vi "Main.vi"(11 "Module Admin":refnum<class "Delacor_lib_QMH_Module Admin.lvclass">) -> ()   [LabVIEW 2020, in "Configuration.lvlib"]
doc: "This template is based off of the Queued Message Handler design pattern and the Queued Message Handler project template that ships with LabVIEW.\n\nThe main difference is that the queue is private to this module and communication between modules is performed via Broadcast and Request events.\n\nRequest events are wrapped in public API methods and are handled in the Event Handling Loop (EHL) of this VI. Any module can register for Broadcast events sent by this module. The EHL generates messages based on user interface actions.\n\nThe Message Handling Loop (MHL) processes messages generated by the EHL, or by other messages. The messages are string values, so new messages can be added easily to the Message Cases case structure in the MHL. Each message cluster can also provide an optional value for Message Data, which is a variant that can be converted to whatever message-specific data is required.\n_____\nBased on DQMH Project Template 6.1.0.94."
uses:
  Configuration.lvlib
  <vilib>/Delacor/Delacor QMH/Libraries/Module Admin_class/Delacor_lib_QMH_Module Admin.lvclass
  Module Data--cluster.ctl
  <vilib>/Delacor/Delacor QMH/Libraries/Message Queue_class/Delacor_lib_QMH_Message Queue.lvclass/Delacor_lib_QMH_Message Queue.ctl
  Stop Argument--cluster.ctl
  <vilib>/Delacor/Delacor QMH/Libraries/Module Admin_class/Delacor_lib_QMH_Module Admin.lvclass/Delacor_lib_QMH_Module Admin.ctl
  Write config Argument--cluster.ctl
  Config data.ctl
  Set config path Argument--cluster.ctl
  Load config Argument--cluster.ctl
  Load config (Reply Payload)--cluster.ctl
  <vilib>/Utility/miscctls.llb/LVPointTypeDef.ctl
  <vilib>/Delacor/Delacor QMH/Libraries/Message Queue_class/Delacor_lib_QMH_Enqueue Message (Single).vi
  <vilib>/Delacor/Delacor QMH/Libraries/Module Admin_class/Delacor_lib_QMH_Get External Launch.vi
  <vilib>/Utility/error.llb/Error Cluster From Error Code.vi
  <vilib>/Utility/config.llb/Write Key (Double).vi
  <vilib>/Utility/config.llb/Read Key (Double).vi
  <vilib>/ErrorRing/Error Ring.xnode
  <vilib>/Delacor/Delacor QMH/Libraries/Message Queue_class/Delacor_lib_QMH_Message Queue.lvclass
  <vilib>/Utility/config.llb/Read Key (String).vi
  <vilib>/Utility/config.llb/Write Key (String).vi
  <vilib>/Utility/config.llb/NI_LVConfig.lvlib
panel:
  out "error out":errorcluster
  out "Status":string
  in  "Simulate MHL Error":bool
  in  "Simulate EHL Error":bool
  # "Other QMH Modules communicate with this Module via its Public API (wrappers for its Request Events).\n\nThis Module communicates with other Modules via its Broadcast Events.\nAny module that wants to get these messages, just registers for this module's Broadcast events."
  # "This template is for the Delacor Modified Queued Message Handler design pattern.\n\nSee the block diagram for more information on how to use this template."
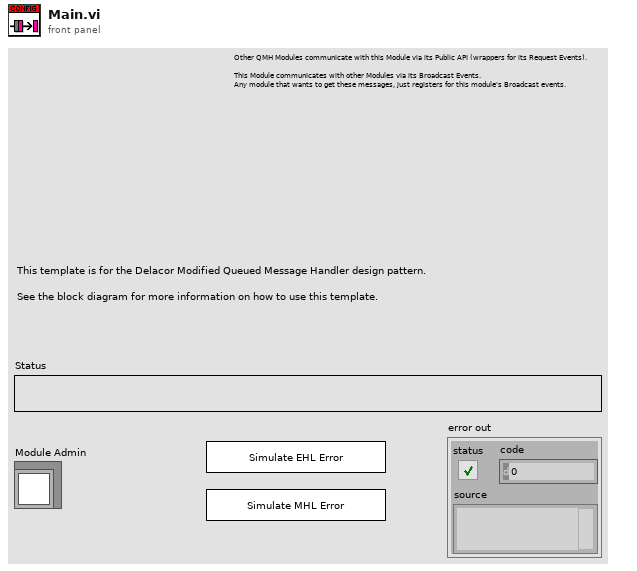
[diagram p1: front panel]
types:
  T1 = typedef "Configuration.lvlib/Request Events--cluster.ctl" = cluster{"Stop Module":refnum<user-event>, "Show Panel":refnum<user-event>, "Hide Panel":refnum<user-event>, "Get Module Execution Status":refnum<user-event>, "Show Diagram":refnum<user-event>, "Write config":refnum<user-event>, "Set config path":refnum<user-event>, "Load config":refnum<user-event>}
  T2 = typedef "Configuration.lvlib/Module Data--cluster.ctl" = cluster{"Status":string, "Config path":path}
  T3 = enum32{"invalid lock state", "Not Locked", "Locked (No Password)", "Password-protected"}
  T4 = typedef "Configuration.lvlib/Stop Argument--cluster.ctl" = cluster{"Origin":string, "Exit via Stop Module Req?":bool, "Wait for Module to stop?":bool}
  T5 = typedef "Configuration.lvlib/Write config Argument--cluster.ctl" = cluster{"Config path":path, "Data":T6}
  T6 = typedef "Configuration.lvlib/Config data.ctl" = cluster{"Arduino":string, "Steps per rev":dbl, "Config path":path, "Pitch":dbl, "Osciloscopio":refnum<visa-resource-name>}
  T7 = typedef "Configuration.lvlib/Set config path Argument--cluster.ctl" = cluster{"Config path":path}
  T8 = typedef "Configuration.lvlib/Load config Argument--cluster.ctl" = cluster{"Wait Notifier":refnum<notifier>, "wait for reply":bool}
  T9 = typedef "LVPointTypeDef.ctl" = cluster{"Horizontal":i16, "Vertical":i16}
  T10 = enum32{"Invalid", "Standard", "Closed", "Hidden", "Minimized", "Maximized"}
  T11 = typedef "Configuration.lvlib/Load config (Reply Payload)--cluster.ctl" = cluster{"Data":T6, "error":errorcluster}
  T12 = typedef "NI_LVConfig.lvlib/Config Data RefNum.ctl" = refnum<k1>
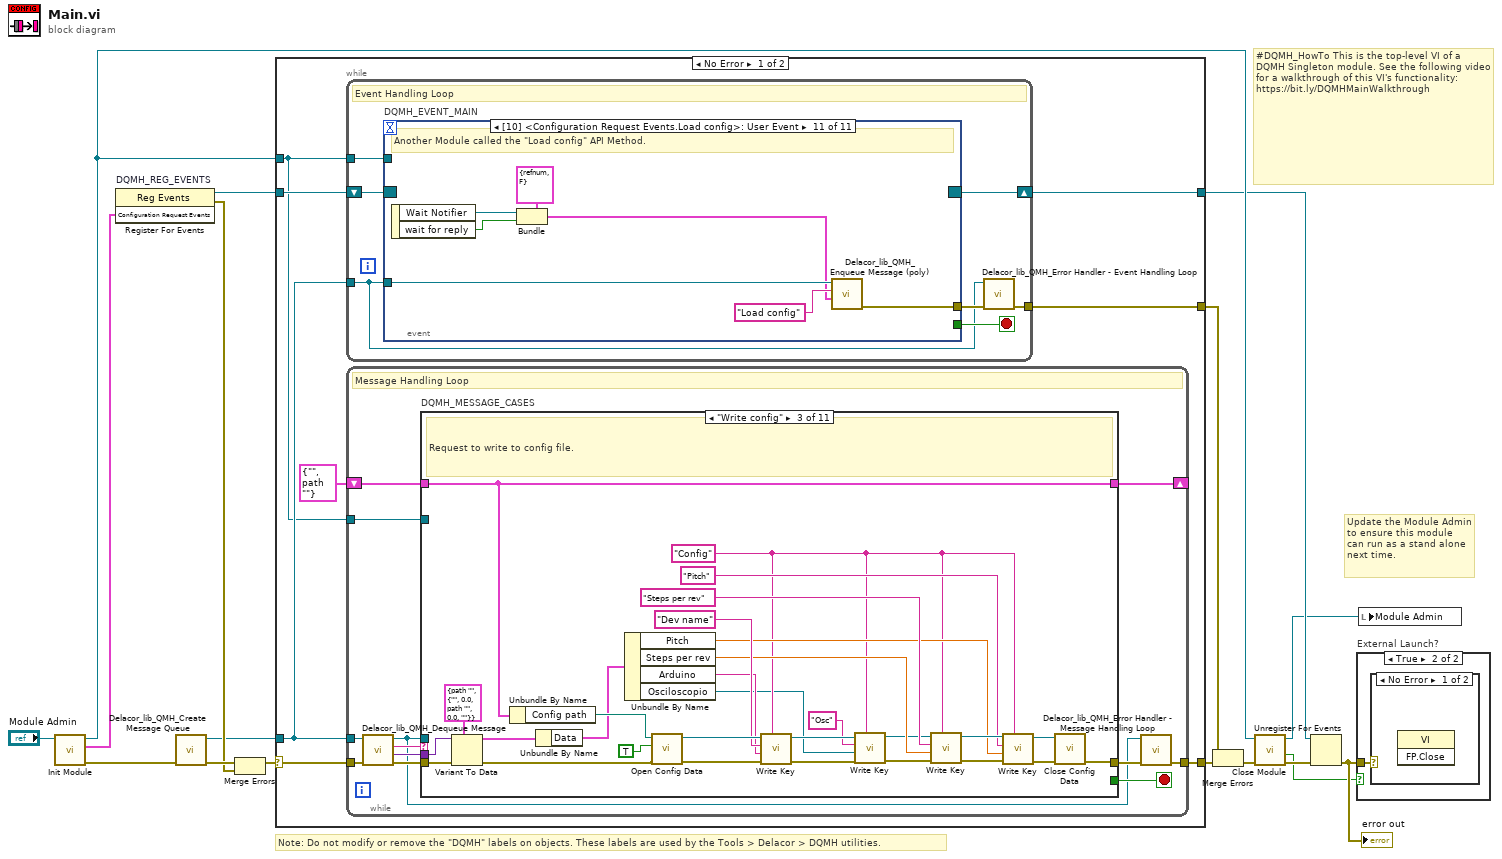
[diagram p0: block diagram]
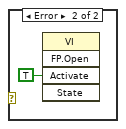
[diagram p3: hidden frame]
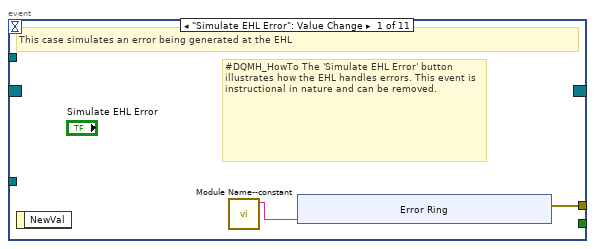
[diagram p4: hidden frame]
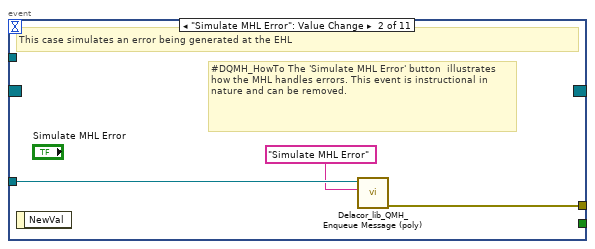
[diagram p5: hidden frame]
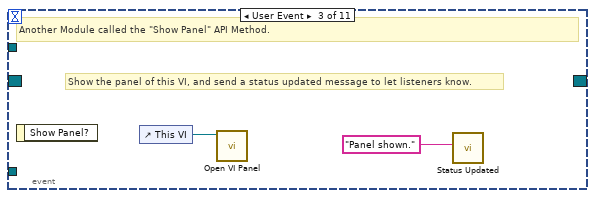
[diagram p6: hidden frame]
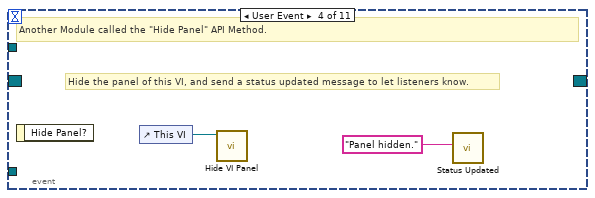
[diagram p7: hidden frame]
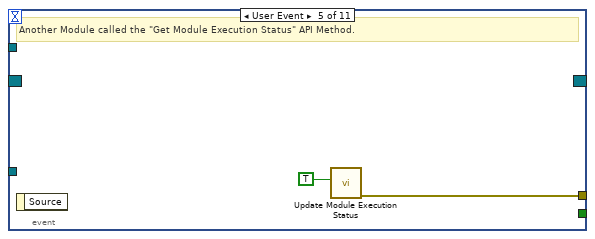
[diagram p8: hidden frame]
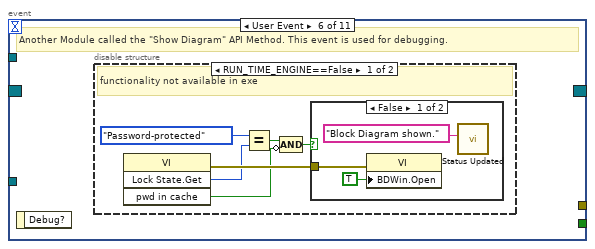
[diagram p9: hidden frame]
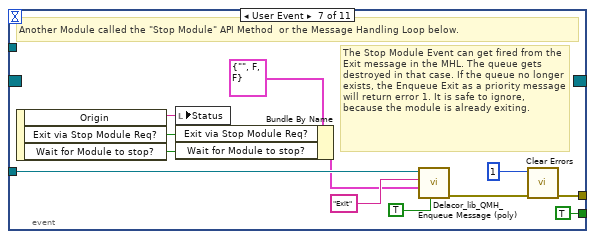
[diagram p12: hidden frame]
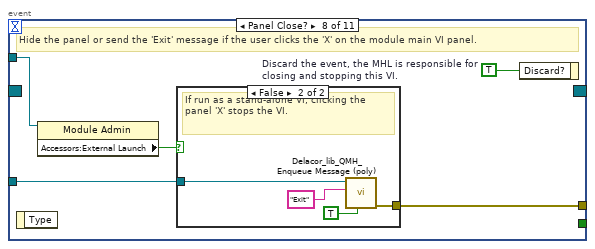
[diagram p13: hidden frame]
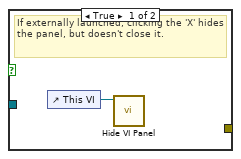
[diagram p14: hidden frame]
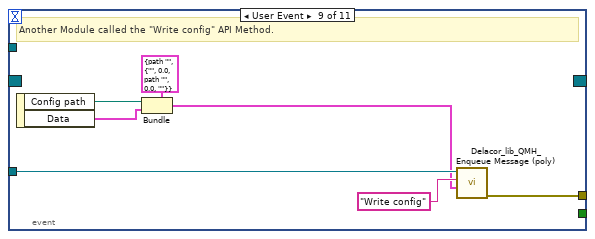
[diagram p15: hidden frame]
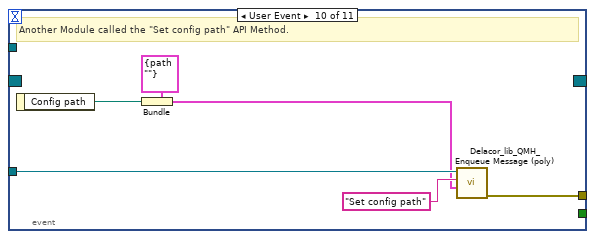
[diagram p16: hidden frame]
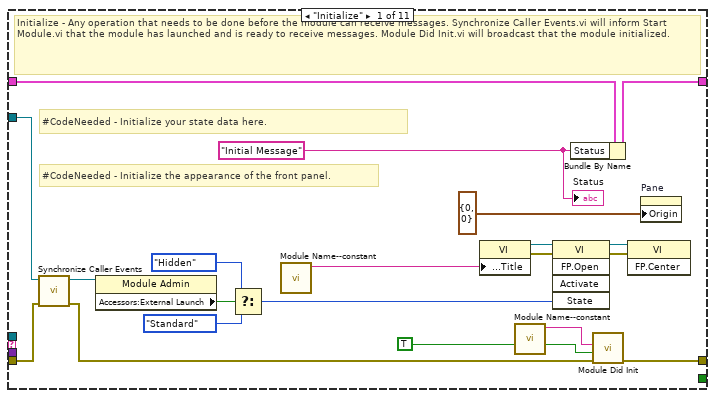
[diagram p17: hidden frame]
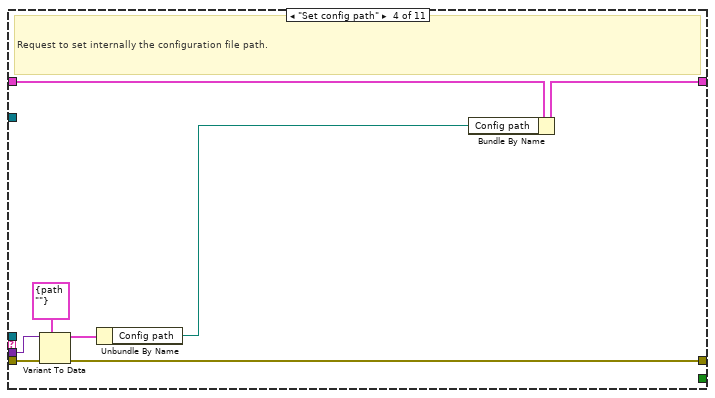
[diagram p19: hidden frame]
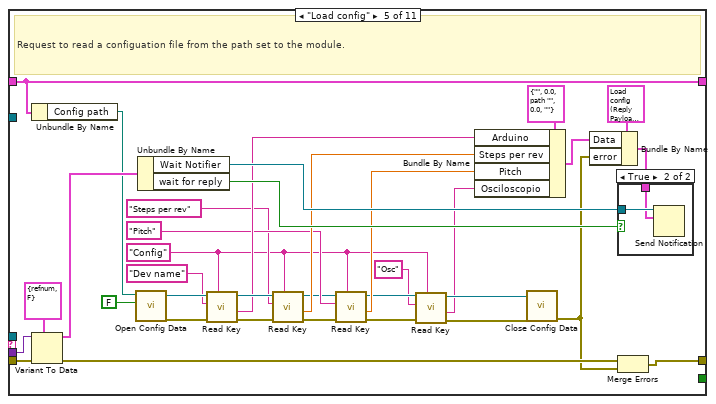
[diagram p20: hidden frame]
diagram:
  # "#DQMH_HowTo This is the top-level VI of a DQMH Singleton module. See the following video for a walkthrough of this VI's functionality: https://bit.ly/DQMHMainWalkthrough"
  # "Note: Do not modify or remove the \"DQMH\" labels on objects. These labels are used by the Tools > Delacor > DQMH utilities."
  # "Update the Module Admin to ensure this module can run as a stand alone next time."
  n1 = call "Init Module.vi"("Singleton Module Admin in"="Module Admin") -> ("error out"=w16:errorcluster, "Configuration Request Events"=w5:T1, "Singleton Module Admin out"=w8:refnum<class "Delacor_lib_QMH_Module Admin.lvclass">)  [unwired: 8 in]
  n2 = register-events "DQMH_REG_EVENTS"(w5) -> (reference out=w6:refnum<event-registration>, error out=w9:errorcluster)  [unwired: 2 in]
  n3 = call <vilib>:"Delacor_lib_QMH_Create Message Queue.vi"("error in"=w16) -> ("error out"=w11:errorcluster, "Message Queue"=w4:refnum<class "Delacor_lib_QMH_Message Queue.lvclass">)  [unwired: 9 in]
  n4 = Merge Errors(w11, w9) -> (w10:errorcluster)
  n5 = case shown="No Error" w10 {
    selector: w10 -> [w23 w274]
    tunnel: [w25 w273] -> w17
    tunnel: [w22 w279] -> w7
    tunnel: w6 -> [w20 w279]
    tunnel: w4 -> [w19 w272]
    tunnel: [w24 _] -> w14
    tunnel: w8 -> [w18 w275]
    frame No Error {
      n6 = while {
        tunnel: w19 -> [w26]
        shift-right: [w29] -> w22
        shift-left: w20 -> [w30]
        tunnel: [w31] -> w24
        tunnel: w18 -> [w27]
        stop <- w28 stop-if-true
        # "Event Handling Loop"
        n7 = event "DQMH_EVENT_MAIN" shown="[10] <Configuration Request Events.Load config>: User Event" {
          selector: w30 -> [_ _ _ _ _ _ _ _ _ _ _]
          dyn-events: [_ _ _ _ _ _ _ _ _ _ _] -> w29
          timeout: _ -> [_ _ _ _ _ _ _ _ _ _ _]
          tunnel: [_ _ _ _ _ _ TRUE ("Discard?") _ _ _ _] -> w28
          tunnel: w26 -> [_ w43 _ _ _ _ w67 w74 w88 w94 w101]
          tunnel: [w34 w44 _ _ w50 _ w70 w76 w84 w89 w95] -> w32
          tunnel: w27 -> [_ _ _ _ _ _ _ w73 _ _ _]
          event "Simulate EHL Error": Value Change {
            # "#DQMH_HowTo The 'Simulate EHL Error' button  illustrates how the EHL handles errors. This event is instructional in nature and can be removed."
            # "This case simulates an error being generated at the EHL"
            n8 = event-data() -> ()  [unwired: 1 in, 1 out]
            n9 = call "Module Name--constant.vi"() -> ("Module Name"=w33:string)  [unwired: 11 in]
            n10 = xnode "Error Ring"("parameter 0"=w33) -> ("error out"=w34:errorcluster)
          }
          event "Simulate MHL Error": Value Change {
            # "#DQMH_HowTo The 'Simulate MHL Error' button  illustrates how the MHL handles errors. This event is instructional in nature and can be removed."
            # "This case simulates an error being generated at the EHL"
            n11 = event-data() -> ()  [unwired: 1 in, 1 out]
            n12 = call-poly <vilib>:"Delacor_lib_QMH_Enqueue Message (poly).vi"("Message"="Simulate MHL Error", "Message Queue in"=w43) -> ("error out"=w44:errorcluster)  [unwired: 8 in, 1 out]
          }
          event User Event {
            # "Show the panel of this VI, and send a status updated message to let listeners know."
            # "Another Module called the \"Show Panel\" API Method."
            n13 = event-data() -> ()  [unwired: 1 in, 1 out]
            n14 = control-ref of="This VI"() -> (w46:refnum<vi>)
            n15 = call "Open VI Panel.vi"("VI"=w46) -> ()  [unwired: 10 in, 1 out]
            n16 = call "Status Updated.vi"("Status"="Panel shown." ("format string")) -> ()  [unwired: 10 in, 1 out]
          }
          event User Event {
            # "Hide the panel of this VI, and send a status updated message to let listeners know."
            # "Another Module called the \"Hide Panel\" API Method."
            n17 = event-data() -> ()  [unwired: 1 in, 1 out]
            n18 = control-ref of="This VI"() -> (w48:refnum<vi>)
            n19 = call "Hide VI Panel.vi"("VI"=w48) -> ()  [unwired: 10 in, 1 out]
            n20 = call "Status Updated.vi"("Status"="Panel hidden." ("format string")) -> ()  [unwired: 10 in, 1 out]
          }
          event User Event {
            # "Another Module called the \"Get Module Execution Status\" API Method."
            n21 = event-data() -> ()  [unwired: 1 in, 1 out]
            n22 = call "Update Module Execution Status.vi"("Running?"=TRUE) -> ("error out"=w50:errorcluster)  [unwired: 10 in]
          }
          event User Event {
            # "Another Module called the \"Show Diagram\" API Method. This event is used for debugging."
            n23 = event-data() -> ()  [unwired: 1 in, 1 out]
            n24 = disable-structure shown="RUN_TIME_ENGINE==False" {
              frame condition #0 (active) {
                # "functionality not available in exe"
                n25 = invoke class="VI" method="Lock State.Get"() -> (error out=w56:errorcluster, "Get Lock State"=w55:T3, "pwd in cache"=w52:bool)  [unwired: 4 in, 1 out]
                n26 = Equal?(x=T3."Password-protected", y=w55) -> (x = y?=w53:bool)
                n27 = Compound Arithmetic op=AND(w53, invert w52) -> (w51:bool)
                n28 = case shown="False" w51 {
                  tunnel: w56 -> [w59 _]
                  frame False {
                    n29 = property class="VI"(error in=w59, "BDWin.Open"=TRUE ("Block Diagram Window:Open")) -> ()  [unwired: 1 in, 2 out]
                    n30 = call "Status Updated.vi"("Status"="Block Diagram shown." ("format string")) -> ()  [unwired: 10 in, 1 out]
                  }
                  frame True {
                    # "Password-protected VI, and the password is not in the cache. Do not show the diagram."
                  }
                }
              }
              frame condition #1 {
              }
            }
          }
          event User Event {
            # "The Stop Module Event can get fired from the Exit message in the MHL. The queue gets destroyed in that case. If the queue no longer exists, the Enqueue Exit as a priority message will return error 1. It is safe to ignore, because the module is already exiting."
            # "Another Module called the \"Stop Module\" API Method  or the Message Handling Loop below."
            n31 = event-data() -> ("Origin"=w66:string, "Exit via Stop Module Req?"=w62:bool, "Wait for Module to stop?"=w61:bool)  [unwired: 1 in]
            n32 = local write "Status"(w66) -> ()
            n33 = Bundle By Name(cluster=T4 {"Origin"="", "Exit via Stop Module Req?"=FALSE, "Wait for Module to stop?"=FALSE} ("Stop Argument"), "Exit via Stop Module Req?"=w62, "Wait for Module to stop?"=w61) -> (w60:T4)
            n34 = call-poly <vilib>:"Delacor_lib_QMH_Enqueue Message (poly).vi"("Priority Message? (F)"=TRUE, "Message Data"=w60, "Message"="Exit", "Message Queue in"=w67) -> ("error out"=w71:errorcluster)  [unwired: 6 in, 1 out]
            n35 = call <vilib>:"Clear Errors.vi"("error in (no error)"=w71, "specific error code to clear (0: all)"=1) -> ("error out"=w70:errorcluster)  [unwired: 4 in, 1 out]
          }
          event Panel Close? {
            w75 = TRUE  # Discard the event, the MHL is responsible for closing and stopping this VI.
            # "Hide the panel or send the 'Exit' message if the user clicks the 'X' on the module main VI panel."
            n36 = event-data() -> ()  [unwired: 1 in, 1 out]
            n37 = property class="Module Admin"(reference=w73) -> ("Accessors:External Launch"=w72:bool)  [unwired: 1 in, 2 out]
            n38 = case shown="False" w72 {
              tunnel: w74 -> [_ w80]
              tunnel: [_ w81] -> w76
              frame True {
                # "If externally launched, clicking the 'X' hides the panel, but doesn't close it."
                n39 = control-ref of="This VI"() -> (w77:refnum<vi>)
                n40 = call "Hide VI Panel.vi"("VI"=w77) -> ()  [unwired: 10 in, 1 out]
              }
              frame False {
                # "If run as a stand-alone VI, clicking the panel 'X' stops the VI."
                n41 = call-poly <vilib>:"Delacor_lib_QMH_Enqueue Message (poly).vi"("Priority Message? (F)"=TRUE, "Message"="Exit", "Message Queue in"=w80) -> ("error out"=w81:errorcluster)  [unwired: 7 in, 1 out]
              }
            }
            n42 = event-data("Discard?"=w75) -> ()  [unwired: 1 in, 1 out]
          }
          event User Event {
            # "Another Module called the \"Write config\" API Method."
            n43 = event-data() -> ("Config path"=w83:path, "Data"=w82:T6)  [unwired: 1 in]
            n44 = Bundle(cluster=T5 {"Config path"=path "", "Data"={"Arduino"="", "Steps per rev"=0.0, "Config path"=path "", "Pitch"=0.0, "Osciloscopio"=""}} ("Write config Argument"), "Config path"=w83, "Data"=w82) -> (w85:T5)
            n45 = call-poly <vilib>:"Delacor_lib_QMH_Enqueue Message (poly).vi"("Message Data"=w85, "Message"="Write config", "Message Queue in"=w88) -> ("error out"=w84:errorcluster)  [unwired: 7 in, 1 out]
          }
          event User Event {
            # "Another Module called the \"Set config path\" API Method."
            n46 = event-data() -> ("Config path"=w90:path)  [unwired: 1 in]
            n47 = Bundle(cluster=T7 {"Config path"=path ""} ("Set config path Argument"), "Config path"=w90) -> (w91:T7)
            n48 = call-poly <vilib>:"Delacor_lib_QMH_Enqueue Message (poly).vi"("Message Data"=w91, "Message"="Set config path", "Message Queue in"=w94) -> ("error out"=w89:errorcluster)  [unwired: 7 in, 1 out]
          }
          event User Event {
            # "Another Module called the \"Load config\" API Method."
            n49 = event-data() -> ("Wait Notifier"=w97:refnum<notifier>, "wait for reply"=w96:bool)  [unwired: 1 in]
            n50 = Bundle(cluster=T8 {"Wait Notifier"=refnum, "wait for reply"=FALSE} ("Load config Argument"), "Wait Notifier"=w97, "wait for reply"=w96) -> (w98:T8)
            n51 = call-poly <vilib>:"Delacor_lib_QMH_Enqueue Message (poly).vi"("Message Data"=w98, "Message"="Load config", "Message Queue in"=w101) -> ("error out"=w95:errorcluster)  [unwired: 7 in, 1 out]
          }
        }
        n52 = call-dynamic "Delacor_lib_QMH_Error Handler - Event Handling Loop.vi"("error in"=w32, "Message Queue in"=w26) -> ("dup error in"=w31:errorcluster)  [unwired: 8 in, 1 out]
      }
      n53 = while {
        tunnel: w19 -> [w104]
        shift-right: [w108] -> _
        shift-left: T2 {"Status"="", "Config path"=path ""} ("Data Cluster") -> [w109]
        tunnel: w23 -> [w112]
        tunnel: [w110] -> w25
        tunnel: w18 -> [w102]
        stop <- w107 stop-if-true
        # "Message Handling Loop"
        n54 = call-dynamic "Delacor_lib_QMH_Dequeue Message.vi"("error in"=w112, "Message Queue in"=w104) -> ("error out"=w111:errorcluster, "Message Data"=w105:variant, "Message"=w106:string, "Message Queue out"=w103:refnum<class "Delacor_lib_QMH_Message Queue.lvclass">)  [unwired: 6 in]
        n55 = case "DQMH_MESSAGE_CASES" shown="\"Write config\"" w106 {
          selector: w106 -> [_ _ _ _ _ _ _ _ _ _ w259]
          tunnel: w103 -> [_ _ _ _ _ _ _ _ w229 w251 _]
          tunnel: w111 -> [w131 w135 w164 w172 w207 w212 w214 w219 w236 w257 w261]
          tunnel: [w129 w135 w149 w171 w199 w211 w214 w218 w232 w254 w262] -> w113
          tunnel: w109 -> [w120 w134 w160 w167 w198 w210 w213 w216 w231 w250 w260]
          tunnel: [w119 w134 w160 w165 w198 w210 w213 w216 w231 w250 w260] -> w108
          tunnel: [_ _ _ _ _ _ _ _ _ w249 _] -> w107
          tunnel: w105 -> [_ _ w163 w170 w206 _ _ _ w230 w248 _]
          tunnel: w102 -> [w121 _ _ _ _ _ _ _ w228 w243 _]
          frame "Initialize" {
            w115 = "Initial Message" ("Initial Message")
            # "#CodeNeeded - Initialize the appearance of the front panel."
            # "#CodeNeeded - Initialize your state data here."
            # "Initialize - Any operation that needs to be done before the module can receive messages. Synchronize Caller Events.vi will inform Start Module.vi that the module has launched and is ready to receive messages. Module Did Init.vi will broadcast that the module initialized."
            n56 = call "Synchronize Caller Events.vi"("error in (no error)"=w131, "Singleton Module Admin in"=w121) -> ("error out"=w130:errorcluster, "Singleton Module Admin out"=w116:refnum<class "Delacor_lib_QMH_Module Admin.lvclass">)  [unwired: 8 in]
            n57 = property class="Module Admin"(reference=w116) -> ("Accessors:External Launch"=w125:bool)  [unwired: 1 in, 2 out]
            n58 = Select(t=T10."Hidden" ("State"), s=w125, f=T10."Standard" ("State")) -> (s? t:f=w122:T10)
            n59 = call "Module Name--constant.vi"() -> ("Module Name"=w128:string)  [unwired: 11 in]
            n60 = property class="VI"("Front Panel.Title"=w128) -> (reference out=w127:refnum<vi>, error out=w133:errorcluster)  [unwired: 2 in]
            n61 = call "Module Name--constant.vi"() -> ("Module Name"=w117:string)  [unwired: 11 in]
            n62 = invoke class="VI" method="FP.Open"(reference=w127, error in=w133, "State"=w122) -> (reference out=w126:refnum<vi>, error out=w132:errorcluster)  [unwired: 2 in, 3 out]
            n63 = Bundle By Name(cluster=w120, "Status"=w115) -> (w119:T2)
            n64 = call "Module Did Init.vi"("error in (no error)"=w130, "Initialized?"=TRUE, "Origin"=w117) -> ("error out"=w129:errorcluster)  [unwired: 8 in]
            n65 = invoke class="VI" method="FP.Center"(reference=w126, error in=w132) -> ()  [unwired: 1 in, 3 out]
            n66 = property on="Pane" class="Pane"("Origin"=T9 {"Horizontal"=0, "Vertical"=0}) -> ()  [unwired: 2 in, 2 out]
            "Status" <- w115
          }
          frame "---Module Specific---" {
            # "Separator -- The following cases handle messages specific to this Module."
          }
          frame "Write config" {
            w138 = "Config" ("section")
            # "Request to write to config file."
            n67 = Variant To Data(error in=w164, type=T5 {"Config path"=path "", "Data"={"Arduino"="", "Steps per rev"=0.0, "Config path"=path "", "Pitch"=0.0, "Osciloscopio"=""}} ("Write config Argument"), Variant=w163) -> (data=w161:T5, error out=w159:errorcluster)
            n68 = Unbundle By Name(w160) -> ("Config path"=w158:path)
            n69 = Unbundle By Name(w161) -> ("Data"=w153:T6)
            n70 = Unbundle By Name(w153) -> ("Pitch"=w143:dbl, "Steps per rev"=w150:dbl, "Arduino"=w152:string, "Osciloscopio"=w136:refnum<visa-resource-name>)
            n71 = call <vilib>:"Open Config Data.vi"("error in (no error)"=w159, "create file if necessary (T)"=TRUE, "configuration file path"=w158) -> ("error out"=w156:errorcluster, "refnum"=w155:T12)  [unwired: 6 in, 1 out]
            n72 = call-poly <vilib>:"Write Key.vi"("section"=w138, "error in (no error)"=w156, "value"=w152, "key"="Dev name", "refnum"=w155) -> ("error out"=w140:errorcluster, "refnum out"=w142:T12)  [unwired: 4 in, 1 out]
            n73 = call-poly <vilib>:"Write Key.vi"("section"=w138, "error in (no error)"=w140, "value"=w136, "key"="Osc", "refnum"=w142) -> ("error out"=w139:errorcluster, "refnum out"=w141:T12)  [unwired: 4 in, 1 out]
            n74 = call-poly <vilib>:"Write Key.vi"("section"=w138, "error in (no error)"=w139, "value"=w150, "key"="Steps per rev", "refnum"=w141) -> ("error out"=w148:errorcluster, "refnum out"=w146:T12)  [unwired: 4 in, 1 out]
            n75 = call-poly <vilib>:"Write Key.vi"("section"=w138, "error in (no error)"=w148, "value"=w143, "key"="Pitch", "refnum"=w146) -> ("error out"=w147:errorcluster, "refnum out"=w145:T12)  [unwired: 4 in, 1 out]
            n76 = call <vilib>:"Close Config Data.vi"("error in (no error)"=w147, "refnum"=w145) -> ("error out"=w149:errorcluster)  [unwired: 8 in, 1 out]
          }
          frame "Set config path" {
            # "Request to set internally the configuration file path."
            n77 = Variant To Data(error in=w172, type=T7 {"Config path"=path ""} ("Set config path Argument"), Variant=w170) -> (data=w168:T7, error out=w171:errorcluster)
            n78 = Unbundle By Name(w168) -> ("Config path"=w166:path)
            n79 = Bundle By Name(cluster=w167, "Config path"=w166) -> (w165:T2)
          }
          frame "Load config" {
            w175 = "Config" ("section")
            # "Request to read a configuation file from the path set to the module."
            n80 = Unbundle By Name(w198) -> ("Config path"=w197:path)
            n81 = Variant To Data(error in=w207, type=T8 {"Wait Notifier"=refnum, "wait for reply"=FALSE} ("Load config Argument"), Variant=w206) -> (data=w204:T8, error out=w196:errorcluster)
            n82 = call <vilib>:"Open Config Data.vi"("create file if necessary (T)"=FALSE, "configuration file path"=w197) -> ("error out"=w193:errorcluster, "refnum"=w194:T12)  [unwired: 7 in, 1 out]
            n83 = Unbundle By Name(w204) -> ("Wait Notifier"=w203:refnum<notifier>, "wait for reply"=w202:bool)
            n84 = call-poly <vilib>:"Read Key.vi"("section"=w175, "error in (no error)"=w193, "key"="Dev name", "refnum"=w194) -> ("error out"=w191:errorcluster, "value"=w188:string, "refnum out"=w190:T12)  [unwired: 4 in, 1 out]
            n85 = call-poly <vilib>:"Read Key.vi"("section"=w175, "error in (no error)"=w191, "key"="Steps per rev", "refnum"=w190) -> ("error out"=w184:errorcluster, "value"=w187:dbl, "refnum out"=w181:T12)  [unwired: 4 in, 1 out]
            n86 = call-poly <vilib>:"Read Key.vi"("section"=w175, "error in (no error)"=w184, "key"="Pitch" ("section"), "refnum"=w181) -> ("error out"=w179:errorcluster, "value"=w180:dbl, "refnum out"=w177:T12)  [unwired: 4 in, 1 out]
            n87 = call-poly <vilib>:"Read Key.vi"("section"=w175, "error in (no error)"=w179, "key"="Osc", "refnum"=w177) -> ("error out"=w178:errorcluster, "value"=w173:string, "refnum out"=w176:T12)  [unwired: 4 in, 1 out]
            n88 = Bundle By Name(cluster=T6 {"Arduino"="", "Steps per rev"=0.0, "Config path"=path "", "Pitch"=0.0, "Osciloscopio"=""} ("Data"), "Arduino"=w188, "Steps per rev"=w187, "Pitch"=w180, "Osciloscopio"=w173) -> (w186:T6)
            n89 = call <vilib>:"Close Config Data.vi"("error in (no error)"=w178, "refnum"=w176) -> ("error out"=w185:errorcluster)  [unwired: 8 in, 1 out]
            n90 = Bundle By Name(cluster=T11 {"Data"={"Arduino"="", "Steps per rev"=0.0, "Config path"=path "", "Pitch"=0.0, "Osciloscopio"=""}, "error"={"status"=FALSE, "code"=0, "source"=""}} ("Load config (Reply Payload)"), "Data"=w186, "error"=w185) -> (w201:T11)
            n91 = case shown="True" w202 {
              tunnel: w203 -> [_ w209]
              tunnel: w201 -> [_ w208]
              frame False {
              }
              frame True {
                n92 = Send Notification(notification=w208, notifier=w209) -> ()  [unwired: 1 in, 2 out]
              }
            }
            n93 = Merge Errors(w196, w185) -> (w199:errorcluster)
          }
          frame "---Copy This Frame---" {
            # "Duplicate this frame when creating new messages.  Change this comment in the duplicated frame to describe this message."
            n94 = Merge Errors(w212) -> (w211:errorcluster)
          }
          frame "---Exit and Error Handling---" {
            # "Separator - The following cases handle errors and exit messages."
          }
          frame "Simulate MHL Error" {
            # "#DQMH_HowTo The 'Simulate MHL Error' button  illustrates how the MHL handles errors. This event is instructional in nature and can be removed."
            # "Simulate an error occurring at the MHL"
            n95 = call "Module Name--constant.vi"() -> ("Module Name"=w215:string)  [unwired: 11 in]
            n96 = xnode "Error Ring"("parameter 0"=w215) -> ("error out"=w217:errorcluster)
            n97 = Merge Errors(w219, w217) -> (w218:errorcluster)
          }
          frame "Error" {
            # "#CodeRecommended - If you ever change the name of this \"Error\" message, you'll need to update the name in the Check Loop Error.vi as well."
            # "#CodeRecommended - If the module is running in standalone mode (External Launch = FALSE), this code will pop up an error dialog and call the 'Exit' message if an error occurs. Add more fine-grained error handling here."
            # "Error - Check the error message data and respond accordingly. This message is sent by the \"Error Handler\" VIs at the end of each loop in this application."
            n98 = property class="Module Admin"(reference=w228) -> ("Accessors:External Launch"=w227:bool)  [unwired: 1 in, 2 out]
            n99 = Variant To Data(error in=w236, type=errorcluster {"status"=FALSE, "code"=0, "source"=""} ("error constant"), Variant=w230) -> (data=w237:errorcluster, error out=w234:errorcluster)
            n100 = call "Error Reported.vi"("Error"=w237) -> ()  [unwired: 10 in, 1 out]
            n101 = case shown="False" w227 {
              tunnel: [w242 _] -> w233
              tunnel: w229 -> [w240 _]
              tunnel: w237 -> [w241 _]
              frame False {
                # "If the module is running standalone, then pop up an error dialog and call the \"Exit\" message."
                n102 = call <vilib>:"Simple Error Handler.vi"("error in (no error)"=w241) -> ()  [unwired: 4 in, 5 out]
                n103 = call-poly <vilib>:"Delacor_lib_QMH_Enqueue Message (poly).vi"("Priority Message? (F)"=TRUE, "Message"="Exit", "Message Queue in"=w240) -> ("error out"=w242:errorcluster)  [unwired: 7 in, 1 out]
              }
              frame True {
                # "If the module was launched externally, calling the Error Reported broadcast VI is the only action performed by the \"Error\" message. The module's caller can then process the error appropriately."
              }
            }
            n104 = Merge Errors(w234, w233) -> (w232:errorcluster)
            n105 = local write "error out"(w232) -> ()
          }
          frame "Exit" {
            w247 = 91  # 91: not all Exit messages will have an argument
            w249 = TRUE  # Stop the VI
            # "Release the message queue reference"
            # "#CodeNeeded - Add any required cleanup code here"
            # "Exit - Exit the application."
            n106 = Variant To Data(error in=w257, type=T4 {"Origin"="", "Exit via Stop Module Req?"=FALSE, "Wait for Module to stop?"=FALSE} ("Stop Argument"), Variant=w248) -> (data=w245:T4, error out=w253:errorcluster)
            n107 = call <vilib>:"Clear Errors.vi"("error in (no error)"=w253, "specific error code to clear (0: all)"=w247) -> ("error out"=w256:errorcluster)  [unwired: 4 in, 1 out]
            n108 = control-ref of="This VI"() -> (w244:refnum<vi>)
            n109 = call-dynamic "Delacor_lib_QMH_Release Message Queue.vi"("error in"=w256, "Message Queue"=w251) -> ("error out"=w255:errorcluster)  [unwired: 9 in]
            n110 = call "Handle Exit.vi"("Stop Argument"=w245, "Admin in"=w243, "VI reference"=w244) -> ("error out"=w252:errorcluster)  [unwired: 7 in, 1 out]
            n111 = Merge Errors(w255, w252) -> (w254:errorcluster)
          }
          frame Default {
            # "'Default' case only runs if there is a message that isn't defined in any of the other cases.  Output a programming error."
            n112 = call "Module Name--constant.vi"() -> ("Module Name"=w258:string)  [unwired: 11 in]
            n113 = xnode "Error Ring"("parameter 0"=w259, "parameter 1"=w258) -> ("error out"=w263:errorcluster)
            n114 = Merge Errors(w261, w263) -> (w262:errorcluster)
          }
        }
        n115 = call-dynamic "Delacor_lib_QMH_Error Handler - Message Handling Loop.vi"("error in"=w113, "Message Queue in"=w103) -> ("dup error in"=w110:errorcluster)  [unwired: 8 in, 1 out]
      }
    }
    frame Error {
      # "Synchronize Caller Events.vi will inform Start Module.vi that the module has launched and will let the code calling Start Module.vi register for broadcasts and would permit the caller receive the broadcast that an error occurred at launch time."
      n116 = call-dynamic "Delacor_lib_QMH_Release Message Queue.vi"("error in"=w274, "Message Queue"=w272) -> ("error out"=w273:errorcluster)  [unwired: 9 in]
      n117 = call "Synchronize Caller Events.vi"("Singleton Module Admin in"=w275) -> ("error out"=w280:errorcluster)  [unwired: 9 in, 1 out]
      n118 = call "Module Name--constant.vi"() -> ("Module Name"=w278:string)  [unwired: 11 in]
      n119 = Format Into String(format string="An error occurred during initialization. %s is no longer running.", w278) -> (resulting string=w276:string)  [unwired: 2 in, 1 out]
      n120 = Merge Errors(w273, w280) -> (w281:errorcluster)
      n121 = call "Error Reported.vi"("Additional Information"=w276, "Error"=w281) -> ()  [unwired: 9 in, 1 out]
    }
  }
  n122 = Merge Errors(w14, w17) -> (w13:errorcluster)
  n123 = call "Close Module.vi"("error in (no error)"=w13, "Module Admin in"=w8) -> ("error out"=w15:errorcluster, "External Launch"=w1:bool, "Module Admin out"=w2:refnum<class "Delacor_lib_QMH_Module Admin.lvclass">)  [unwired: 7 in]
  n124 = Unregister For Events(event registration refnum=w7, error in=w15) -> (error out=w12:errorcluster)
  "error out" <- w12
  n125 = case "External Launch?" shown="True" w1 {
    tunnel: w12 -> [_ w282]
    frame False {
    }
    frame True {
      n126 = case shown="No Error" w282 {
        frame No Error {
          n127 = invoke class="VI" method="FP.Close"() -> ()  [unwired: 3 in, 3 out]
        }
        frame Error {
          n128 = invoke class="VI" method="FP.Open"("Activate"=TRUE ("Activate?")) -> ()  [unwired: 4 in, 5 out]
        }
      }
    }
  }
  n129 = local write "Module Admin"(w2) -> ()
